vi "GetText.vi"(8 "error in":errorcluster, 11 "cRIO in":refnum<class "can port.lvclass">) -> (0 "error out":errorcluster, 1 "additional text":string, 2 "text":string, 3 "cRIO out":refnum<class "can port.lvclass">, 4 "glyph":string)   [LabVIEW 2013, in "can port.lvclass"]
uses:
  can port.lvclass
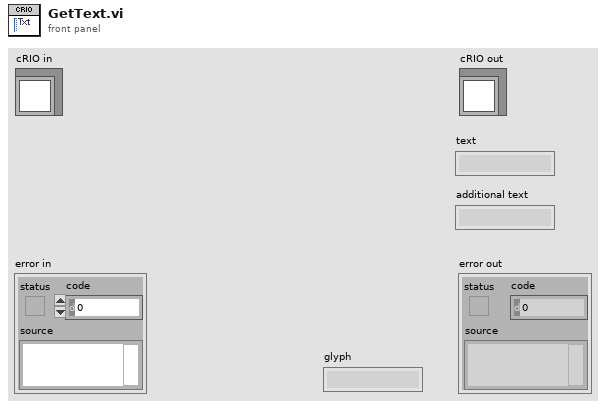
[diagram p1: front panel]
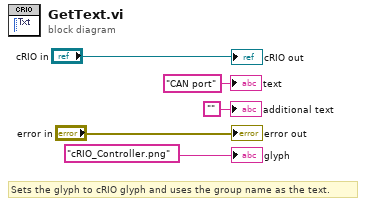
[diagram p0: block diagram]
diagram:
  # "Sets the glyph to cRIO glyph and uses the group name as the text."
  "error out" <- "error in"
  "cRIO out" <- "cRIO in"
  "text" <- "CAN port" ("text")
  "additional text" <- ""
  "glyph" <- "cRIO_Controller.png" ("glyph")
